vi "Phasor Update Gate Parameters Visibility v2.vi"(7 "Edit User-defined Gate":refnum<vi>, 8 "error in (no error)":errorcluster, 11 "Gate Parameters in":refnum<vi>) -> (0 "error out":errorcluster, 2 "Gate Parameters":T1={"First Gate Start"=0.0, "Use Gate Center"=FALSE, "Gate Width"=0.0, "Gate Step"=0.0, "# Gates"=1.0, "Gate Type"=enum."Square", "Edge Width"=0.0, "Top Slope"=0.0, "Reversed Sawtooth?"=FALSE, "Analytical Computation"=FALSE, "Integration"=enum."Item 0", "Tolerance"=1.0, "# Steps"=1.0, "Type of User-defined Function"=enum."Gate", "Use Gate Step"=FALSE} {"# Steps" min=0.0; "Tolerance" min=0.0; "Top Slope" min=0.0; "Edge Width" min=0.0; "Gate Step" min=0.0; "# Gates" min=1.0 step=1.0; "Gate Width" min=0.0}, 3 "Phasor Explorer Gate Parameters out":refnum<vi>)   [LabVIEW 2021, in "Phasor.lvlib"]
doc: "Updates gate parameters visibility."
uses:
  Phasor.lvlib
  Phasor Explorer Gate Parameters.ctl
  Phasor Gate Type.ctl
  Phasor Type of User-defined Function.ctl
  Phasor Explorer.lvlib
panel:
  out "Same # Elements?":bool
  out "Labels":string[](array[string])
  in  "Type of User-defined Function":T3
  # "see the AlliGator License on the block diagram (Ctrl+E or Window:Show Block Diagram)"
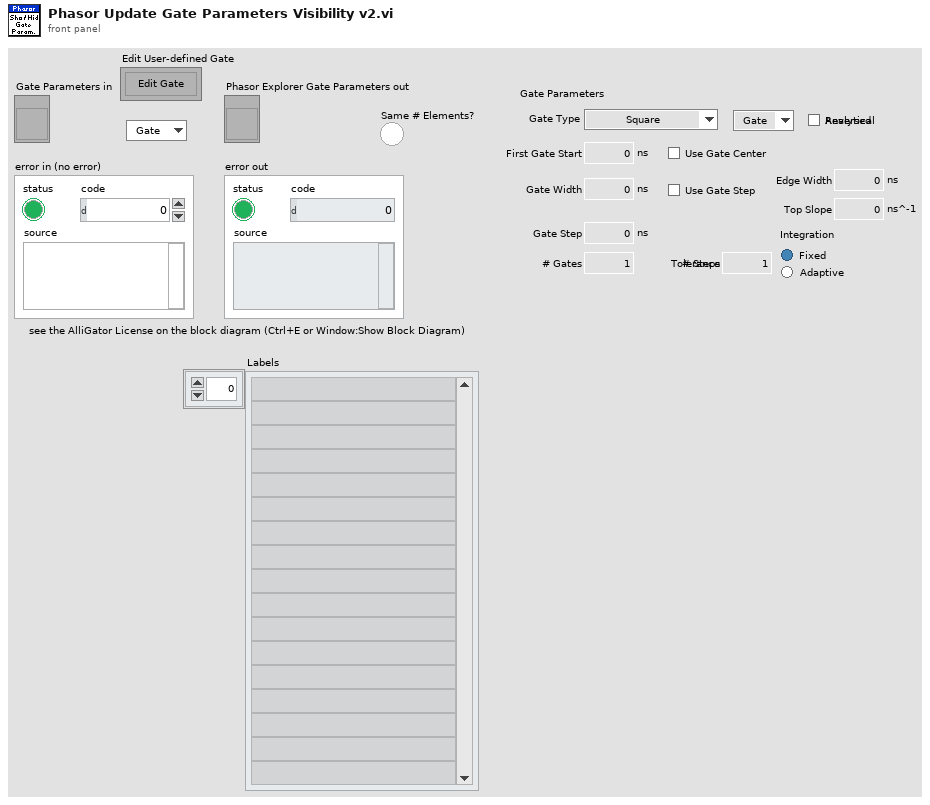
[diagram p1: front panel]
types:
  T1 = typedef "Phasor Explorer.lvlib/Phasor Explorer Gate Parameters.ctl" = cluster{"First Gate Start":dbl[unit], "Use Gate Center":bool, "Gate Width":dbl[unit], "Gate Step":dbl[unit], "# Gates":dbl, "Gate Type":T2, "Edge Width":dbl[unit], "Top Slope":dbl[unit], "Reversed Sawtooth?":bool, "Analytical Computation":bool, "Integration":enum32{"Item 0", "Item 1"}, "Tolerance":dbl, "# Steps":dbl, "Type of User-defined Function":T3, "Use Gate Step":bool}
  T2 = typedef "Phasor.lvlib/Phasor Gate Type.ctl" = enum16{"Square", "Finite Edge Square", "Finite Edge, Tilted Top Square", "Triangle", "Sawtooth", "User-defined"}
  T3 = typedef "Phasor.lvlib/Phasor Type of User-defined Function.ctl" = enum16{"Gate", "IRF"}
  T4 = typedef "Phasor Explorer Gate Parameters.ctl" = cluster{"First Gate Start":dbl[unit], "Use Gate Center":bool, "Gate Width":dbl[unit], "Gate Step":dbl[unit], "# Gates":dbl, "Gate Type":T5, "Edge Width":dbl[unit], "Top Slope":dbl[unit], "Reversed Sawtooth?":bool, "Analytical Computation":bool, "Integration":enum32{"Item 0", "Item 1"}, "Tolerance":dbl, "# Steps":dbl, "Type of User-defined Function":T6, "Use Gate Step":bool}
  T5 = typedef "Gate Type.ctl" = enum16{"Square", "Finite Edge Square", "Finite Edge, Tilted Top Square", "Triangle", "Sawtooth", "User-defined"}
  T6 = typedef "Type of User-defined Function.ctl" = enum16{"Gate", "IRF"}
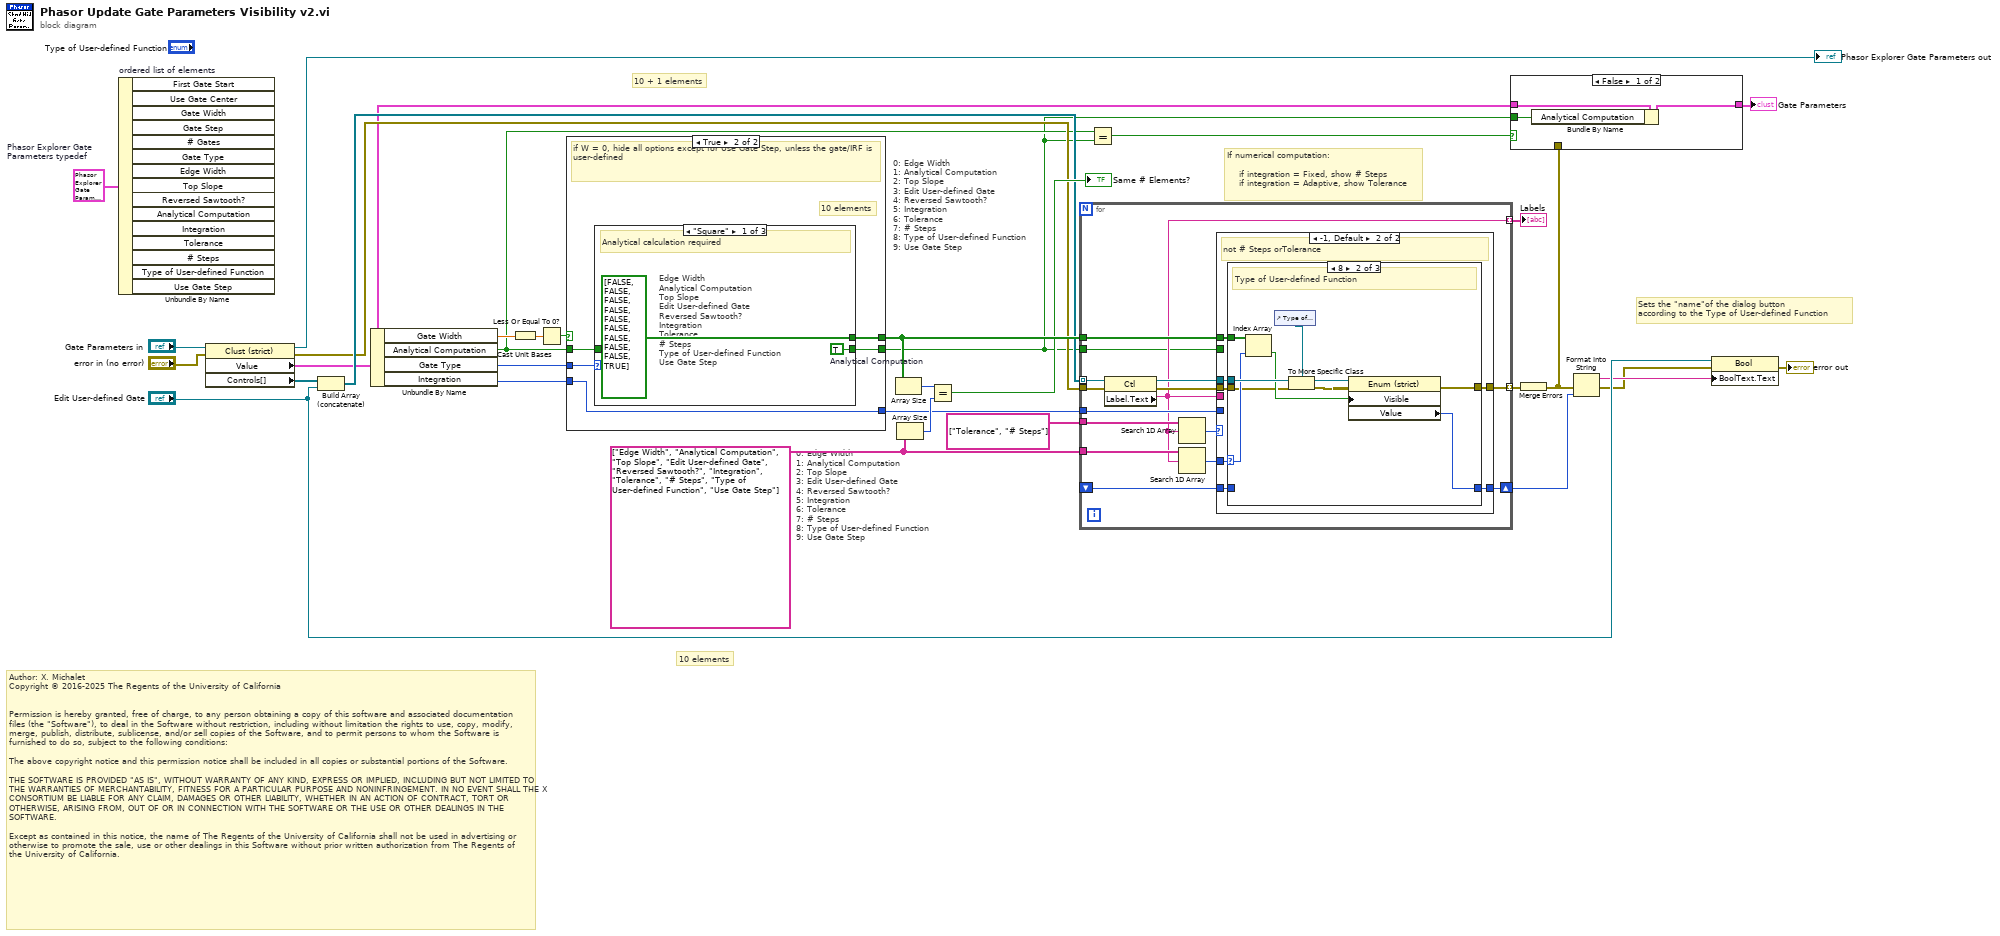
[diagram p0: block diagram]
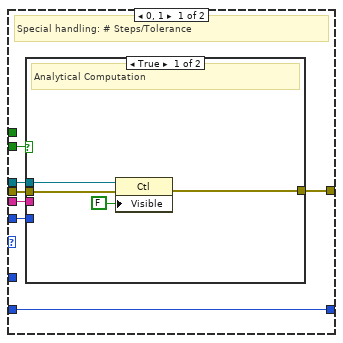
[diagram p3: hidden frame]
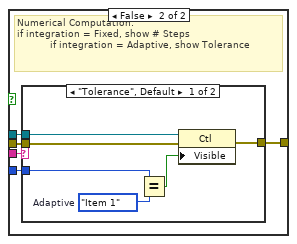
[diagram p4: hidden frame]
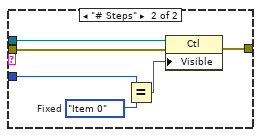
[diagram p5: hidden frame]
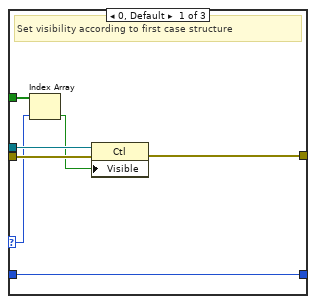
[diagram p6: hidden frame]
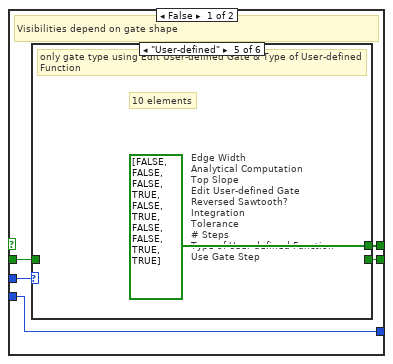
[diagram p8: hidden frame]
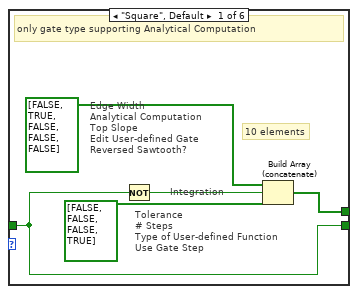
[diagram p9: hidden frame]
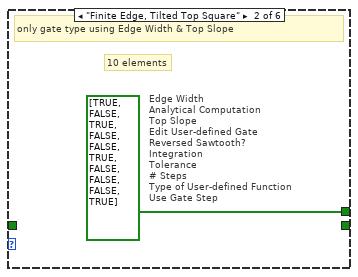
[diagram p10: hidden frame]
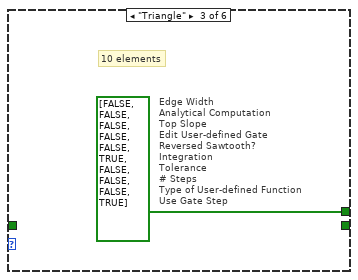
[diagram p11: hidden frame]
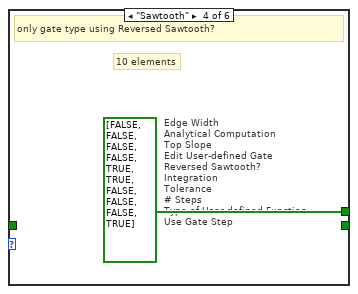
[diagram p12: hidden frame]
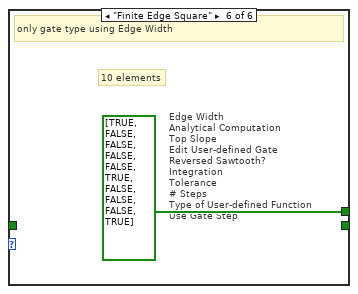
[diagram p13: hidden frame]
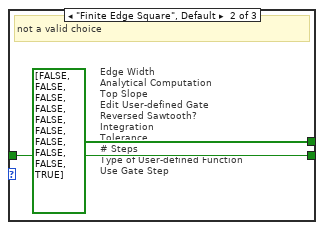
[diagram p14: hidden frame]
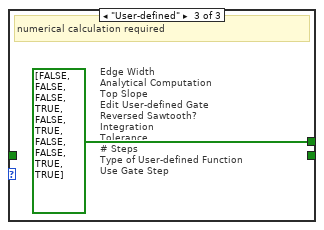
[diagram p15: hidden frame]
diagram:
  w21 = T1 {"First Gate Start"=0.0, "Use Gate Center"=FALSE, "Gate Width"=0.0, "Gate Step"=0.0, "# Gates"=1.0, "Gate Type"=enum."Square", "Edge Width"=0.0, "Top Slope"=0.0, "Reversed Sawtooth?"=FALSE, "Analytical Computation"=FALSE, "Integration"=enum."Item 0", "Tolerance"=1.0, "# Steps"=1.0, "Type of User-defined Function"=enum."Gate", "Use Gate Step"=FALSE}  # Phasor Explorer Gate Parameters typedef
  w17 = string[] ["Edge Width", "Analytical Computation", "Top Slope", "Edit User-defined Gate", "Reversed Sawtooth?", "Integration", "Tolerance", "# Steps", "Type of User-defined Function", "Use Gate Step"] ("Label.Text")
  # "Author: X. Michalet\nCopyright © 2016-2025 The Regents of the University of California\n \n\nPermission is hereby granted, free of charge, to any person obtaining a copy of this software and associated documentation files (the \"Software\"), to deal in the Software without restriction, including without limitation the rights to use, copy, modify, merge, publish, distribute, sublicense, and/or sell copies of the Software, and to permit persons to whom the Software is furnished to do so, subject to the following conditions:\n\nThe above copyright notice and this permission notice shall be included in all copies or substantial portions of the Software.\n\nTHE SOFTWARE IS PROVIDED \"AS IS\", WITHOUT WARRANTY OF ANY KIND, EXPRESS OR IMPLIED, INCLUDING BUT NOT LIMITED TO THE WARRANTIES OF MERCHANTABILITY, FITNESS FOR A PARTICULAR PURPOSE AND NONINFRINGEMENT. IN NO EVENT SHALL THE X CONSORTIUM BE LIABLE FOR ANY CLAIM, DAMAGES OR OTHER LIABILITY, WHETHER IN AN ACTION OF CONTRACT, TORT OR OTHERWISE, ARISING FROM, OUT OF OR IN CONNECTION WITH THE SOFTWARE OR THE USE OR OTHER DEALINGS IN THE SOFTWARE.\n\nExcept as contained in this notice, the name of The Regents of the University of California shall not be used in advertising or otherwise to promote the sale, use or other dealings in this Software without prior written authorization from The Regents of the University of California."
  # "10 + 1 elements"
  # "0: Edge Width\n1: Analytical Computation\n2: Top Slope\n3: Edit User-defined Gate\n4: Reversed Sawtooth?\n5: Integration\n6: Tolerance\n7: # Steps\n8: Type of User-defined Function\n9: Use Gate Step"
  # "Sets the \"name\"of the dialog button\naccording to the Type of User-defined Function"
  # "If numerical computation:\n\n    if integration = Fixed, show # Steps\n    if integration = Adaptive, show Tolerance"
  # "0: Edge Width\n1: Analytical Computation\n2: Top Slope\n3: Edit User-defined Gate\n4: Reversed Sawtooth?\n5: Integration\n6: Tolerance\n7: # Steps\n8: Type of User-defined Function\n9: Use Gate Step"
  # "10 elements"
  n1 = Unbundle By Name "ordered list of elements"(w21) -> ()  [unwired: 15 out]
  n2 = property class="Clust (strict)"(reference="Gate Parameters in", error in="error in (no error)") -> (reference out=→"Phasor Explorer Gate Parameters out":refnum<vi>, error out=w12:errorcluster, "Value"=w4:T4, "Controls[]"=w30:refnum<vi>[])
  n3 = Build Array (concatenate)(w30, "Edit User-defined Gate") -> (w13:refnum<vi>[])
  n4 = Unbundle By Name(w4) -> ("Gate Width"=w8:dbl[unit], "Analytical Computation"=w7:bool, "Gate Type"=w11:T5, "Integration"=w10:enum32{"Item 0", "Item 1"})
  n5 = Cast Unit Bases(0:w8) -> (2:w28:dbl)  [unwired: 1 in]
  n6 = Less Or Equal To 0?(x=w28) -> (x <= 0?=w27:bool)
  n7 = case shown="True" w27 {
    tunnel: [w37 w52] -> w18
    tunnel: [w34 w50] -> w9
    tunnel: w11 -> [w36 w51]
    tunnel: w7 -> [w35 w48]
    tunnel: w10 -> [w34 w50]
    tunnel: [w33 w49] -> w5
    frame False {
      # "Visibilities depend on gate shape"
      n8 = case shown="\"User-defined\"" w36 {
        tunnel: [w41 bool[] [TRUE, FALSE, TRUE, FALSE, FALSE, TRUE, FALSE, FALSE, FALSE, TRUE] ("Label.Text") bool[] [FALSE, FALSE, FALSE, FALSE, FALSE, TRUE, FALSE, FALSE, FALSE, TRUE] ("Label.Text") bool[] [FALSE, FALSE, FALSE, FALSE, TRUE, TRUE, FALSE, FALSE, FALSE, TRUE] ("Label.Text") bool[] [FALSE, FALSE, FALSE, TRUE, FALSE, TRUE, FALSE, FALSE, TRUE, TRUE] ("Label.Text") bool[] [TRUE, FALSE, FALSE, FALSE, FALSE, TRUE, FALSE, FALSE, FALSE, TRUE] ("Label.Text")] -> w37
        tunnel: w35 -> [w38 _ _ _ _ _]
        tunnel: [w38 _ _ _ _ _] -> w33
        frame "Square", Default {
          # "10 elements"
          # "Integration"
          # "Tolerance\n# Steps\nType of User-defined Function\nUse Gate Step"
          # "Edge Width\nAnalytical Computation\nTop Slope\nEdit User-defined Gate\nReversed Sawtooth?"
          # "only gate type supporting Analytical Computation"
          n9 = Not(x=w38) -> (.not. x?=w40:bool)
          n10 = Build Array (concatenate)(bool[] [FALSE, TRUE, FALSE, FALSE, FALSE] ("Label.Text"), w40, bool[] [FALSE, FALSE, FALSE, TRUE] ("Label.Text")) -> (w41:bool[])
        }
        frame "Finite Edge, Tilted Top Square" {
          # "10 elements"
          # "Edge Width\nAnalytical Computation\nTop Slope\nEdit User-defined Gate\nReversed Sawtooth?\nIntegration\nTolerance\n# Steps\nType of User-defined Function\nUse Gate Step"
          # "only gate type using Edge Width & Top Slope"
        }
        frame "Triangle" {
          # "10 elements"
          # "Edge Width\nAnalytical Computation\nTop Slope\nEdit User-defined Gate\nReversed Sawtooth?\nIntegration\nTolerance\n# Steps\nType of User-defined Function\nUse Gate Step"
        }
        frame "Sawtooth" {
          # "10 elements"
          # "Edge Width\nAnalytical Computation\nTop Slope\nEdit User-defined Gate\nReversed Sawtooth?\nIntegration\nTolerance\n# Steps\nType of User-defined Function\nUse Gate Step"
          # "only gate type using Reversed Sawtooth?"
        }
        frame "User-defined" {
          # "10 elements"
          # "Edge Width\nAnalytical Computation\nTop Slope\nEdit User-defined Gate\nReversed Sawtooth?\nIntegration\nTolerance\n# Steps\nType of User-defined Function\nUse Gate Step"
          # "only gate type using Edit User-defined Gate & Type of User-defined Function"
        }
        frame "Finite Edge Square" {
          # "10 elements"
          # "Edge Width\nAnalytical Computation\nTop Slope\nEdit User-defined Gate\nReversed Sawtooth?\nIntegration\nTolerance\n# Steps\nType of User-defined Function\nUse Gate Step"
          # "only gate type using Edge Width"
        }
      }
    }
    frame True {
      # "10 elements"
      # "if W = 0, hide all options except for Use Gate Step, unless the gate/IRF is user-defined"
      n11 = case shown="\"Square\"" w51 {
        tunnel: [bool[] [FALSE, FALSE, FALSE, FALSE, FALSE, FALSE, FALSE, FALSE, FALSE, TRUE] ("Label.Text") bool[] [FALSE, FALSE, FALSE, FALSE, FALSE, FALSE, FALSE, FALSE, FALSE, TRUE] ("Label.Text") bool[] [FALSE, FALSE, FALSE, TRUE, FALSE, TRUE, FALSE, FALSE, TRUE, TRUE] ("Label.Text")] -> w52
        tunnel: [w53 w55 _] -> w49
        tunnel: w48 -> [_ w55 _]
        frame "Square" {
          w53 = TRUE  # Analytical Computation
          # "Edge Width\nAnalytical Computation\nTop Slope\nEdit User-defined Gate\nReversed Sawtooth?\nIntegration\nTolerance\n# Steps\nType of User-defined Function\nUse Gate Step"
          # "Analytical calculation required"
        }
        frame "Finite Edge Square", Default {
          # "Edge Width\nAnalytical Computation\nTop Slope\nEdit User-defined Gate\nReversed Sawtooth?\nIntegration\nTolerance\n# Steps\nType of User-defined Function\nUse Gate Step"
          # "not a valid choice"
        }
        frame "User-defined" {
          # "Edge Width\nAnalytical Computation\nTop Slope\nEdit User-defined Gate\nReversed Sawtooth?\nIntegration\nTolerance\n# Steps\nType of User-defined Function\nUse Gate Step"
          # "numerical calculation required"
        }
      }
    }
  }
  n12 = Array Size(array=w18) -> (size(s)=w16:i32)
  n13 = Array Size(array=w17) -> (size(s)=w15:i32)
  n14 = Equal?(x=w16, y=w15) -> (x = y?=→"Same # Elements?":bool)
  n15 = for {
    tunnel: w17 -> [w72]
    tunnel: w13 -> [w71] mode=indexing
    tunnel: w12 -> [w70]
    tunnel: w18 -> [w69]
    tunnel: [w67] -> w29 mode=indexing
    shift-right: [w64] -> w24
    shift-left: _ -> [w63]
    tunnel: w9 -> [w62]
    tunnel: string[] ["Tolerance", "# Steps"] ("Label.Text") -> [w61]
    tunnel: [w59] -> w19 mode=indexing
    tunnel: w5 -> [w58]
    n16 = property class="Ctl"(reference=w71, error in=w70) -> (reference out=w66:refnum<vi>, error out=w65:errorcluster, "Label.Text"=w59:string)
    n17 = Search 1D Array(1D array=w61, element=w59) -> (index of element=w60:i32)  [unwired: 1 in]
    n18 = Search 1D Array(1D array=w72, element=w59) -> (index of element=w68:i32)  [unwired: 1 in]
    n19 = case shown="-1, Default" w60 {
      tunnel: w69 -> [_ w107]
      tunnel: w68 -> [_ w106]
      tunnel: [w79 w105] -> w67
      tunnel: w66 -> [w78 w104]
      tunnel: w65 -> [w77 w103]
      tunnel: w58 -> [w75 _]
      tunnel: [w76 w102] -> w64
      tunnel: w63 -> [w76 w101]
      tunnel: w62 -> [w73 _]
      tunnel: w59 -> [w74 _]
      frame 0, 1 {
        # "Special handling: # Steps/Tolerance"
        n20 = case shown="True" w75 {
          tunnel: [w83 w88] -> w79
          tunnel: w78 -> [w82 w87]
          tunnel: w77 -> [w81 w86]
          tunnel: w74 -> [_ w85]
          tunnel: w73 -> [_ w84]
          frame True {
            # "Analytical Computation"
            n21 = property class="Ctl"(reference=w82, error in=w81, "Visible"=FALSE) -> (error out=w83:errorcluster)  [unwired: 1 out]
          }
          frame False {
            # "Numerical Computation:\nif integration = Fixed, show # Steps\n           if integration = Adaptive, show Tolerance"
            n22 = case shown="\"Tolerance\", Default" w85 {
              tunnel: [w94 w100] -> w88
              tunnel: w87 -> [w93 w99]
              tunnel: w86 -> [w92 w98]
              tunnel: w84 -> [w91 w97]
              frame "Tolerance", Default {
                w90 = enum32{"Item 0", "Item 1"}."Item 1"  # Adaptive
                n23 = Equal?(x=w91, y=w90) -> (x = y?=w89:bool)
                n24 = property class="Ctl"(reference=w93, error in=w92, "Visible"=w89) -> (error out=w94:errorcluster)  [unwired: 1 out]
              }
              frame "# Steps" {
                w96 = enum32{"Item 0", "Item 1"}."Item 0"  # Fixed
                n25 = Equal?(x=w97, y=w96) -> (x = y?=w95:bool)
                n26 = property class="Ctl"(reference=w99, error in=w98, "Visible"=w95) -> (error out=w100:errorcluster)  [unwired: 1 out]
              }
            }
          }
        }
      }
      frame -1, Default {
        # "not # Steps orTolerance"
        n27 = case shown="8" w106 {
          selector: w106 -> [w111 w122 _]
          tunnel: w104 -> [w114 w124 _]
          tunnel: w103 -> [w113 w118 w126]
          tunnel: w107 -> [w112 w123 _]
          tunnel: [w109 w120 w126] -> w105
          tunnel: [w108 w115 w125] -> w102
          tunnel: w101 -> [w108 _ w125]
          frame 0, Default {
            # "Set visibility according to first case structure"
            n28 = Index Array(array=w112, index=w111) -> (element=w110:bool)
            n29 = property class="Ctl"(reference=w114, error in=w113, "Visible"=w110) -> (error out=w109:errorcluster)  [unwired: 1 out]
          }
          frame 8 {
            # "Type of User-defined Function"
            n30 = Index Array(array=w123, index=w122) -> (element=w121:bool)
            n31 = control-ref of="Type of User-defined Function"() -> (w116:refnum<vi>)
            n32 = To More Specific Class(target class=w116, reference=w124, error in=w118) -> (specific class reference=w119:refnum<vi>, error out=w117:errorcluster)
            n33 = property class="Enum (strict)"(reference=w119, error in=w117, "Visible"=w121) -> (error out=w120:errorcluster, "Value"=w115:T6)  [unwired: 1 out]
          }
          frame -1 {
            # "do nothing"
          }
        }
      }
    }
  }
  "Labels" <- w19
  n34 = Equal?(x=w7, y=w5) -> (x = y?=w6:bool)
  n35 = Merge Errors(w29) -> (w3:errorcluster)
  n36 = case shown="False" w6 {
    tunnel: w5 -> [w129 _]
    tunnel: w4 -> [w128 w130]
    tunnel: w3 -> [_ _]
    tunnel: [w127 w130] -> w1
    frame False {
      n37 = Bundle By Name(cluster=w128, "Analytical Computation"=w129) -> (w127:T4)
    }
    frame True {
    }
  }
  "Gate Parameters" <- w1
  n38 = Format Into String(error in=w3, w24) -> (resulting string=w23:string, error out=w22:errorcluster)  [unwired: 2 in]
  n39 = property class="Bool"(reference="Edit User-defined Gate", error in=w22, "BoolText.Text"=w23) -> (error out=→"error out":errorcluster)  [unwired: 1 out]
